vi "change pivot.vi"(8 "error in (no error)":errorcluster, 9 "new pivot center":T1 {"Y" format="%.4g"; "X" format="%.4g"}, 11 "select pivot point":T2) -> (0 "error out":errorcluster)   [LabVIEW 2023]
uses:
  Global odometry.vi
  Global INIT.vi
  ctrl defs/ctrl XY coord.ctl
  ctrl defs/ctrl pivot select.ctl
panel:
  out "recalc mod polar":bool
  out "output pivot center":T1 {"Y" format="%.4g"; "X" format="%.4g"}
  out "Old pivot center":T1 {"Y" format="%.4g"; "X" format="%.4g"}
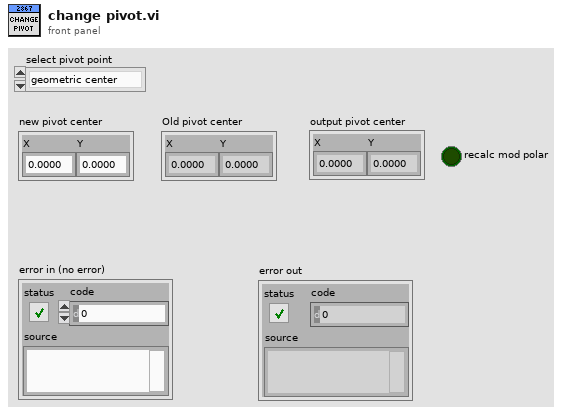
[diagram p1: front panel]
types:
  T1 = typedef "ctrl XY coord.ctl" = cluster{"X":dbl, "Y":dbl}
  T2 = typedef "ctrl pivot select.ctl" = enum16{"geometric center", "CG", "FL", "FR", "RR", "RL", "other"}
  T3 = typedef "ctrl swerve module.ctl" = cluster{"descr":string, "V":dbl, "POS":dbl, "target":dbl, "ABS":dbl, "from pivot to module":cluster{"R":dbl, "theta (deg)":dbl, "theta spin (deg)":dbl}, "coord wrt geom CTR":cluster{"geomX":dbl, "geomY":dbl}, "corner wt (lbm)":dbl}
  T4 = typedef "ctrl robot CG.ctl" = cluster{"mass (lbm)":dbl, "CG":T1, "Zcg":dbl}
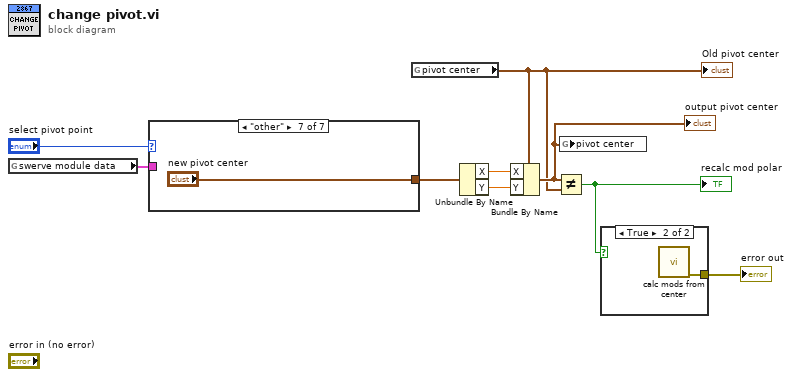
[diagram p0: block diagram]
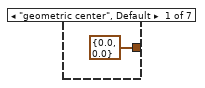
[diagram p3: hidden frame]
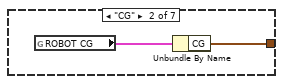
[diagram p4: hidden frame]
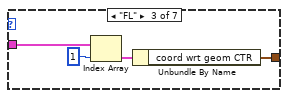
[diagram p5: hidden frame]
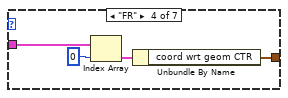
[diagram p6: hidden frame]
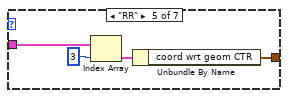
[diagram p7: hidden frame]
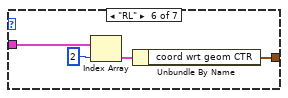
[diagram p8: hidden frame]
diagram:
  n1 = global read "Global odometry.vi" "swerve module data"() -> (w8:T3[])
  n2 = case shown="\"other\"" "select pivot point" {
    tunnel: [T1 {"X"=0.0, "Y"=0.0} ("CG") w11 w13 w17 w22 w25 "new pivot center"] -> w2
    tunnel: w8 -> [_ _ w16 w18 w21 w26 _]
    frame "geometric center", Default {
    }
    frame "CG" {
      n3 = global read "Global INIT.vi" "ROBOT CG"() -> (w12:T4)
      n4 = Unbundle By Name(w12) -> ("CG"=w11:T1)
    }
    frame "FL" {
      n5 = Index Array(array=w16, index=1) -> (element=w14:T3)
      n6 = Unbundle By Name(w14) -> ("coord wrt geom CTR"=w13:cluster{"geomX":dbl, "geomY":dbl})
    }
    frame "FR" {
      n7 = Index Array(array=w18, index=0) -> (element=w19:T3)
      n8 = Unbundle By Name(w19) -> ("coord wrt geom CTR"=w17:cluster{"geomX":dbl, "geomY":dbl})
    }
    frame "RR" {
      n9 = Index Array(array=w21, index=3) -> (element=w23:T3)
      n10 = Unbundle By Name(w23) -> ("coord wrt geom CTR"=w22:cluster{"geomX":dbl, "geomY":dbl})
    }
    frame "RL" {
      n11 = Index Array(array=w26, index=2) -> (element=w27:T3)
      n12 = Unbundle By Name(w27) -> ("coord wrt geom CTR"=w25:cluster{"geomX":dbl, "geomY":dbl})
    }
    frame "other" {
    }
  }
  n13 = global read "Global odometry.vi" "pivot center"() -> (w5:T1)
  "Old pivot center" <- w5
  n14 = Unbundle By Name(w2) -> ("X"=w4:dbl, "Y"=w3:dbl)
  n15 = Bundle By Name(cluster=w5, "X"=w4, "Y"=w3) -> (w6:T1)
  "output pivot center" <- w6
  n16 = Not Equal?(x=w6, y=w5) -> (x != y?=w7:bool)
  "recalc mod polar" <- w7
  n17 = global write "Global odometry.vi" "pivot center"(w6) -> ()
  n18 = case shown="True" w7 {
    tunnel: [_ w30] -> w1
    frame False {
    }
    frame True {
      n19 = call "calc mods from center.vi"() -> ("error out"=w30:errorcluster)  [unwired: 11 in]
    }
  }
  "error out" <- w1
